vi "DataLog Reduce String Offsets.vi"(7 "string offsets":dbl[](array[numeric]), 11 "error in (no error)":errorcluster) -> (6 "reduced offsets":dbl[](array[numeric]), 10 "string indices":dbl[](array[numeric]), 15 "error out":errorcluster)   [LabVIEW 2012]
doc: "Reduces a set of string tag log offsets to two arrays, one containing all unique offsets in ascending order, the other containing indices into this array such that the input array is equivalent to the reduced offsets array indexed at that series indices.\n\nThis allows the number of strings to be read from the tag log to be minimized. This reduces I/O, network, and memory load when performing interactive queries on measurement machines."
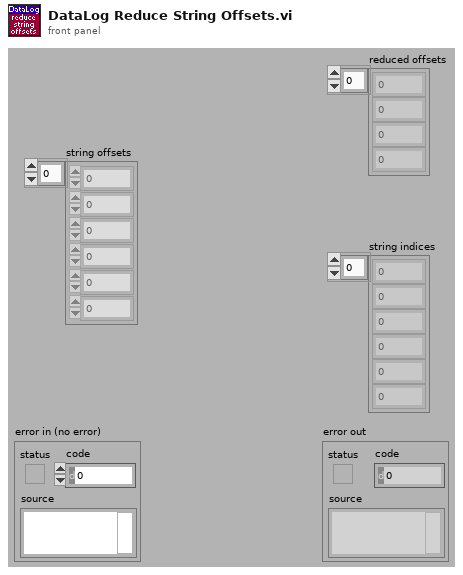
[diagram p1: front panel]
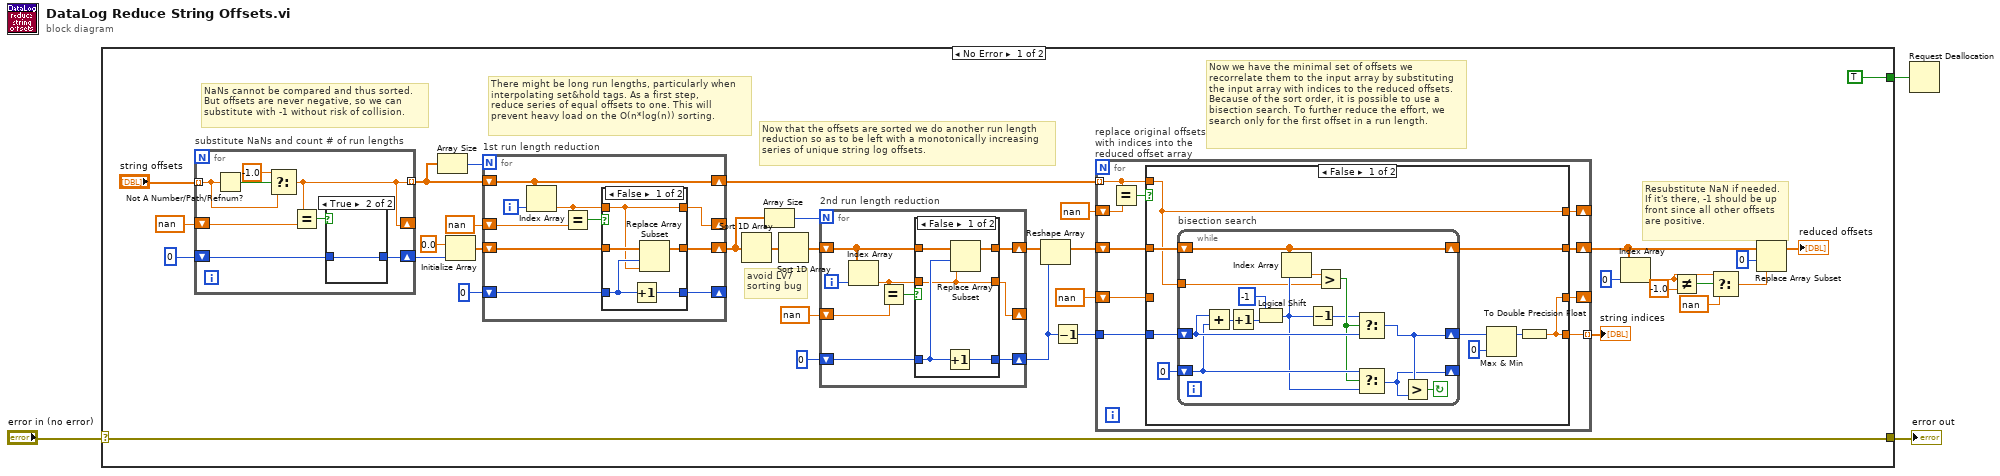
[diagram p0: block diagram]
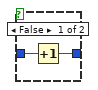
[diagram p5: hidden frame]
diagram:
  n1 = case shown="No Error" "error in (no error)" {
    selector: "error in (no error)" -> [w38 w121]
    tunnel: [w38 w121] -> w2
    tunnel: [TRUE ("flag") _] -> w1
    frame No Error {
      # "Resubstitute NaN if needed.\nIf it's there, -1 should be up\nfront since all other offsets\nare positive."
      # "Now we have the minimal set of offsets we \nrecorrelate them to the input array by substituting\nthe input array with indices to the reduced offsets.\nBecause of the sort order, it is possible to use a\nbisection search. To further reduce the effort, we\nsearch only for the first offset in a run length."
      # "Now that the offsets are sorted we do another run length\nreduction so as to be left with a monotonically increasing\nseries of unique string log offsets."
      # "There might be long run lengths, particularly when\ninterpolating set&hold tags. As a first step,\nreduce series of equal offsets to one. This will\nprevent heavy load on the O(n*log(n)) sorting."
      # "NaNs cannot be compared and thus sorted.\nBut offsets are never negative, so we can\nsubstitute with -1 without risk of collision."
      # "avoid LV7\nsorting bug"
      n2 = for "substitute NaNs and count # of run lengths" {
        tunnel: "string offsets" -> [w115] mode=indexing
        tunnel: [w113] -> w21 mode=indexing
        shift-right: [w113] -> _
        shift-left: nan ("t") -> [w114]
        shift-right: [w110] -> w33
        shift-left: 0 -> [w111]
        n3 = Not A Number/Path/Refnum?(number/path/refnum=w115) -> (NaN/Path/Refnum?=w117:bool)
        n4 = Select(t=-1.0, s=w117, f=w115) -> (s? t:f=w113:dbl)
        n5 = Equal?(x=w113, y=w114) -> (x = y?=w112:bool)
        n6 = case shown="True" w112 {
          tunnel: w111 -> [w119 w120]
          tunnel: [w118 w120] -> w110
          frame False {
            n7 = Increment(x=w119) -> (x+1=w118:i32)
          }
          frame True {
          }
        }
      }
      n8 = Array Size(array=w21) -> (size(s)=w20:i32)
      n9 = Initialize Array(0.0 ("t"), w33) -> (w31:dbl[])
      n10 = for "1st run length reduction" {
        N: w20 -> [_]
        shift-right: [w101] -> w19
        shift-left: w21 -> [w101]
        shift-right: [w96] -> w23
        shift-left: w31 -> [w97]
        shift-right: [w92] -> _
        shift-left: nan ("t") -> [w99]
        shift-right: [w94] -> _
        shift-left: 0 -> [w95]
        i -> [w100]
        n11 = Index Array(array=w101, index=w100) -> (element=w93:dbl)
        n12 = Equal?(x=w93, y=w99) -> (x = y?=w98:bool)
        n13 = case shown="False" w98 {
          tunnel: w97 -> [w105 w109]
          tunnel: [w103 w109] -> w96
          tunnel: w93 -> [w102 w107]
          tunnel: w95 -> [w104 w108]
          tunnel: [w106 w108] -> w94
          tunnel: [w102 w107] -> w92
          frame False {
            n14 = Increment(x=w104) -> (x+1=w106:i32)
            n15 = Replace Array Subset(array=w105, new element=w102, index=w104) -> (w103:dbl[])
          }
          frame True {
          }
        }
      }
      n16 = Sort 1D Array(array=w23) -> (sorted array=w28:dbl[])
      n17 = Array Size(array=w23) -> (size(s)=w22:i32)
      n18 = Sort 1D Array(array=w28) -> (sorted array=w25:dbl[])
      n19 = for "2nd run length reduction" {
        N: w22 -> [_]
        shift-right: [w79] -> _
        shift-left: nan ("t") -> [w83]
        shift-right: [w80] -> w16
        shift-left: 0 -> [w81]
        shift-right: [w75] -> w24
        shift-left: w25 -> [w76]
        i -> [w78]
        n20 = Index Array(array=w76, index=w78) -> (element=w77:dbl)
        n21 = Equal?(x=w77, y=w83) -> (x = y?=w82:bool)
        n22 = case shown="False" w82 {
          tunnel: w77 -> [w85 w90]
          tunnel: w81 -> [w86 w91]
          tunnel: [w88 w91] -> w80
          tunnel: [w85 w90] -> w79
          tunnel: w76 -> [w87 w89]
          tunnel: [w84 w89] -> w75
          frame False {
            n23 = Increment(x=w86) -> (x+1=w88:i32)
            n24 = Replace Array Subset(array=w87, new element=w85, index=w86) -> (w84:dbl[])
          }
          frame True {
          }
        }
      }
      n25 = Reshape Array(w24, w16) -> (w18:dbl[])
      n26 = Decrement(x=w16) -> (x-1=w17:i32)
      n27 = for "replace original offsets with indices into the reduced offset array" {
        tunnel: w19 -> [w43] mode=indexing
        shift-right: [w45] -> w7
        shift-left: w18 -> [w48]
        tunnel: w17 -> [w47]
        tunnel: [w46] -> w15 mode=indexing
        shift-right: [w39] -> _
        shift-left: nan ("t") -> [w44]
        shift-right: [w41] -> _
        shift-left: nan ("t") -> [w40]
        n28 = Equal?(x=w43, y=w44) -> (x = y?=w42:bool)
        n29 = case shown="False" w42 {
          tunnel: w48 -> [w54 w73]
          tunnel: w47 -> [w53 _]
          tunnel: [w50 w74] -> w46
          tunnel: [w51 w73] -> w45
          tunnel: w43 -> [w49 w72]
          tunnel: [w50 w74] -> w41
          tunnel: w40 -> [_ w74]
          tunnel: [w49 w72] -> w39
          frame False {
            n30 = while "bisection search" {
              shift-right: [w63] -> _
              shift-left: 0 -> [w70]
              shift-right: [w69] -> w56
              shift-left: w53 -> [w71]
              tunnel: w49 -> [w60]
              shift-right: [w58] -> w51
              shift-left: w54 -> [w58]
              stop <- w68 continue-if-true
              n31 = Add(x=w71, y=w70) -> (x+y=w66:i32)
              n32 = Increment(x=w66) -> (x+1=w61:i32)
              n33 = Logical Shift(y=-1, x=w61) -> (x << y=w64:i32)
              n34 = Index Array(array=w58, index=w64) -> (element=w59:dbl)
              n35 = Decrement(x=w64) -> (x-1=w62:i32)
              n36 = Greater?(x=w59, y=w60) -> (0:w67:bool)
              n37 = Select(t=w62, s=w67, f=w71) -> (s? t:f=w69:i32)
              n38 = Select(t=w70, s=w67, f=w64) -> (s? t:f=w63:i32)
              n39 = Greater?(x=w69, y=w63) -> (0:w68:bool)
            }
            n40 = Max & Min(x=w56, y=0) -> (max(x,y)=w52:i32)  [unwired: 1 out]
            n41 = To Double Precision Float(number=w52) -> (double precision float=w50:dbl)
          }
          frame True {
          }
        }
      }
      "string indices" <- w15
      n42 = Index Array(array=w7, index=0) -> (element=w9:dbl)
      n43 = Not Equal?(x=w9, y=-1.0) -> (x != y?=w10:bool)
      n44 = Select(t=w9, s=w10, f=nan) -> (s? t:f=w5:dbl)
      n45 = Replace Array Subset(array=w7, new element=w5, index=0) -> (→"reduced offsets":dbl[])
    }
    frame Error {
    }
  }
  "error out" <- w2
  n46 = Request Deallocation(w1) -> ()
